vi "FlexRay_Analyze_signal_values.vi"(10 "TLibFLexRay":T2, 11 "DataBase_array":T1) -> (3 "data out":T3)   [LabVIEW 2014]
uses:
  Typedef/TDBProperties.ctl
  Typedef/TDBECUProperties.ctl
  Typedef/TDBFrameProperties.ctl
  Typedef/CAN/TCANSignal.ctl
  Typedef/LIN/TLINSignal.ctl
  Typedef/FlexRay/TFlexRaySignal.ctl
  Typedef/TDBSignalProperties.ctl
  FlexRay_Function/Typedef/TLibFLexRay.ctl
  Typedef/DataBase_array.ctl
  Typedef/DataBase_array_index.ctl
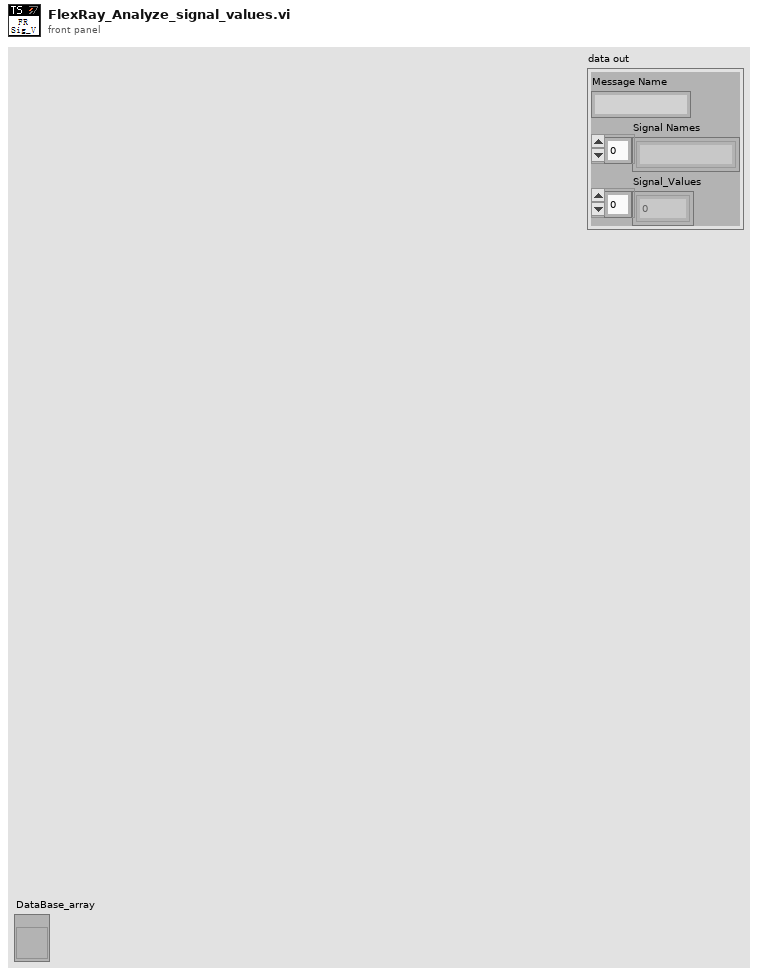
[diagram p1: front panel]
types:
  T1 = typedef "DataBase_array_index.ctl" = refnum<vi>
  T2 = typedef "TLibFLexRay.ctl" = cluster{"FIdxChn":u8, "FChannelMask":u8, "FDir":u8, "FPayloadLength":u8, "FActualPayloadLength":u8, "FCycleNumber":u8, "FCCType":u8, "FFrameType":u8, "FHeaderCRCA":u16, "FHeaderCRCB":u16, "FFrameStateInfo":u16, "FSlotId":u16, "FFrameFlags":u32, "FFrameCRC":u32, "FReserved1":u64, "FReserved2":u64, "FTimeUs":u64, "FData":cluster{"数值":u8, "数值 9":u8, "数值 17":u8, "数值 25":u8, "数值 33":u8, "数值 41":u8, "数值 49":u8, "数值 57":u8, "数值 65":u8, "数值 73":u8, "数值 81":u8, "数值 89":u8, "数值 97":u8, "数值 105":u8, "数值 98":u8, "数值 99":u8, "数值 2":u8, "数值 10":u8, "数值 18":u8, "数值 26":u8, "数值 34":u8, "数值 42":u8, "数值 50":u8, "数值 58":u8, "数值 66":u8, "数值 74":u8, "数值 82":u8, "数值 90":u8, "数值 100":u8, "数值 106":u8, "数值 101":u8, "数值 102":u8, "数值 3":u8, "数值 11":u8, "数值 19":u8, "数值 27":u8, "数值 35":u8, "数值 43":u8, "数值 51":u8, "数值 59":u8, "数值 67":u8, "数值 75":u8, "数值 83":u8, "数值 91":u8, "数值 103":u8, "数值 107":u8, "数值 104":u8, "数值 108":u8, "数值 4":u8, "数值 12":u8, "数值 20":u8, "数值 28":u8, "数值 36":u8, "数值 44":u8, "数值 52":u8, "数值 60":u8, "数值 68":u8, "数值 76":u8, "数值 84":u8, "数值 92":u8, "数值 109":u8, "数值 110":u8, "数值 111":u8, "数值 112":u8, "数值 5":u8, "数值 13":u8, "数值 21":u8, "数值 29":u8, "数值 37":u8, "数值 45":u8, "数值 53":u8, "数值 61":u8, "数值 69":u8, "数值 77":u8, "数值 85":u8, "数值 93":u8, "数值 113":u8, "数值 114":u8, "数值 115":u8, "数值 116":u8, "数值 6":u8, "数值 14":u8, "数值 22":u8, "数值 30":u8, "数值 38":u8, "数值 46":u8, "数值 54":u8, "数值 62":u8, "数值 70":u8, "数值 78":u8, "数值 86":u8, "数值 94":u8, "数值 117":u8, "数值 118":u8, "数值 119":u8, "数值 120":u8, "数值 7":u8, "数值 15":u8, "数值 23":u8, "数值 31":u8, "数值 39":u8, "数值 47":u8, "数值 55":u8, "数值 63":u8, "数值 71":u8, "数值 79":u8, "数值 87":u8, "数值 95":u8, "数值 121":u8, "数值 122":u8, "数值 123":u8, "数值 124":u8, "数值 8":u8, "数值 16":u8, "数值 24":u8, "数值 32":u8, "数值 40":u8, "数值 48":u8, "数值 56":u8, "数值 64":u8, "数值 72":u8, "数值 80":u8, "数值 88":u8, "数值 96":u8, "数值 125":u8, "数值 126":u8, "数值 127":u8, "数值 128":u8, "数值 129":u8, "数值 130":u8, "数值 131":u8, "数值 132":u8, "数值 133":u8, "数值 134":u8, "数值 135":u8, "数值 136":u8, "数值 137":u8, "数值 138":u8, "数值 139":u8, "数值 140":u8, "数值 141":u8, "数值 142":u8, "数值 143":u8, "数值 144":u8, "数值 145":u8, "数值 146":u8, "数值 147":u8, "数值 148":u8, "数值 149":u8, "数值 150":u8, "数值 151":u8, "数值 152":u8, "数值 153":u8, "数值 154":u8, "数值 155":u8, "数值 156":u8, "数值 157":u8, "数值 158":u8, "数值 159":u8, "数值 160":u8, "数值 161":u8, "数值 162":u8, "数值 163":u8, "数值 164":u8, "数值 165":u8, "数值 166":u8, "数值 167":u8, "数值 168":u8, "数值 169":u8, "数值 170":u8, "数值 171":u8, "数值 172":u8, "数值 173":u8, "数值 174":u8, "数值 175":u8, "数值 176":u8, "数值 177":u8, "数值 178":u8, "数值 179":u8, "数值 180":u8, "数值 181":u8, "数值 182":u8, "数值 183":u8, "数值 184":u8, "数值 185":u8, "数值 186":u8, "数值 187":u8, "数值 188":u8, "数值 189":u8, "数值 190":u8, "数值 191":u8, "数值 192":u8, "数值 193":u8, "数值 194":u8, "数值 195":u8, "数值 196":u8, "数值 197":u8, "数值 198":u8, "数值 199":u8, "数值 200":u8, "数值 201":u8, "数值 202":u8, "数值 203":u8, "数值 204":u8, "数值 205":u8, "数值 206":u8, "数值 207":u8, "数值 208":u8, "数值 209":u8, "数值 210":u8, "数值 211":u8, "数值 212":u8, "数值 213":u8, "数值 214":u8, "数值 215":u8, "数值 216":u8, "数值 217":u8, "数值 218":u8, "数值 219":u8, "数值 220":u8, "数值 221":u8, "数值 222":u8, "数值 223":u8, "数值 224":u8, "数值 225":u8, "数值 226":u8, "数值 227":u8, "数值 228":u8, "数值 229":u8, "数值 230":u8, "数值 231":u8, "数值 232":u8, "数值 233":u8, "数值 234":u8, "数值 235":u8, "数值 236":u8, "数值 237":u8, "数值 238":u8, "数值 239":u8, "数值 241":u8, "数值 242":u8, "数值 243":u8, "数值 244":u8, "数值 245":u8, "数值 246":u8, "数值 247":u8, "数值 248":u8, "数值 249":u8, "数值 250":u8, "数值 251":u8, "数值 252":u8, "数值 253":u8, "数值 254":u8, "数值 255":u8}}
  T3 = cluster{"Message Name":string, "Signal Names":string[], "Signal_Values":dbl[]}
  T4 = typedef "DataBase_array.ctl" = cluster{"db_properties":T5, "ECU_array":cluster{"TDBECUProperties":T6, "TX_Frame_array":cluster{"Frame_Properties":T7, "signal_array":T8[]}[], "RX_Frame_array":cluster{"Frame_Properties":T7, "signal_array":T8[]}[]}[]}[]
  T5 = typedef "TDBProperties.ctl" = cluster{"FDBIndex":i32, "FSignalCount":i32, "FFrameCount":i32, "FECUCount":i32, "FSupportedChannelMask":u64, "FName":cluster{"数值":u64, "数值 2":u64, "数值 3":u64, "数值 4":u64, "数值 5":u64, "数值 6":u64, "数值 7":u64, "数值 8":u64, "数值 9":u64, "数值 10":u64, "数值 11":u64, "数值 12":u64, "数值 13":u64, "数值 14":u64, "数值 15":u64, "数值 16":u64, "数值 17":u64, "数值 18":u64, "数值 19":u64, "数值 20":u64, "数值 21":u64, "数值 22":u64, "数值 23":u64, "数值 24":u64, "数值 25":u64, "数值 26":u64, "数值 27":u64, "数值 28":u64, "数值 29":u64, "数值 30":u64, "数值 31":u64, "数值 32":u64, "数值 33":u64, "数值 34":u64, "数值 35":u64, "数值 36":u64, "数值 37":u64, "数值 38":u64, "数值 39":u64, "数值 40":u64, "数值 41":u64, "数值 42":u64, "数值 43":u64, "数值 44":u64, "数值 45":u64, "数值 46":u64, "数值 47":u64, "数值 48":u64, "数值 49":u64, "数值 50":u64, "数值 51":u64, "数值 52":u64, "数值 53":u64, "数值 54":u64, "数值 55":u64, "数值 56":u64, "数值 57":u64, "数值 58":u64, "数值 59":u64, "数值 60":u64, "数值 61":u64, "数值 62":u64, "数值 63":u64, "数值 64":u64}, "FComment":cluster{"数值":u64, "数值 2":u64, "数值 3":u64, "数值 4":u64, "数值 5":u64, "数值 6":u64, "数值 7":u64, "数值 8":u64, "数值 9":u64, "数值 10":u64, "数值 11":u64, "数值 12":u64, "数值 13":u64, "数值 14":u64, "数值 15":u64, "数值 16":u64, "数值 17":u64, "数值 18":u64, "数值 19":u64, "数值 20":u64, "数值 21":u64, "数值 22":u64, "数值 23":u64, "数值 24":u64, "数值 25":u64, "数值 26":u64, "数值 27":u64, "数值 28":u64, "数值 29":u64, "数值 30":u64, "数值 31":u64, "数值 32":u64, "数值 33":u64, "数值 34":u64, "数值 35":u64, "数值 36":u64, "数值 37":u64, "数值 38":u64, "数值 39":u64, "数值 40":u64, "数值 41":u64, "数值 42":u64, "数值 43":u64, "数值 44":u64, "数值 45":u64, "数值 46":u64, "数值 47":u64, "数值 48":u64, "数值 49":u64, "数值 50":u64, "数值 51":u64, "数值 52":u64, "数值 53":u64, "数值 54":u64, "数值 55":u64, "数值 56":u64, "数值 57":u64, "数值 58":u64, "数值 59":u64, "数值 60":u64, "数值 61":u64, "数值 62":u64, "数值 63":u64, "数值 64":u64}, "FFlags":u32, "FDBId":u32}
  T6 = typedef "TDBECUProperties.ctl" = cluster{"FDBIndex":i32, "FECUIndex":i32, "FTxFrameCount":i32, "FRxFrameCount":i32, "FName":cluster{"数值":u64, "数值 2":u64, "数值 3":u64, "数值 4":u64, "数值 5":u64, "数值 6":u64, "数值 7":u64, "数值 8":u64, "数值 9":u64, "数值 10":u64, "数值 11":u64, "数值 12":u64, "数值 13":u64, "数值 14":u64, "数值 15":u64, "数值 16":u64, "数值 17":u64, "数值 18":u64, "数值 19":u64, "数值 20":u64, "数值 21":u64, "数值 22":u64, "数值 23":u64, "数值 24":u64, "数值 25":u64, "数值 26":u64, "数值 27":u64, "数值 28":u64, "数值 29":u64, "数值 30":u64, "数值 31":u64, "数值 32":u64, "数值 33":u64, "数值 34":u64, "数值 35":u64, "数值 36":u64, "数值 37":u64, "数值 38":u64, "数值 39":u64, "数值 40":u64, "数值 41":u64, "数值 42":u64, "数值 43":u64, "数值 44":u64, "数值 45":u64, "数值 46":u64, "数值 47":u64, "数值 48":u64, "数值 49":u64, "数值 50":u64, "数值 51":u64, "数值 52":u64, "数值 53":u64, "数值 54":u64, "数值 55":u64, "数值 56":u64, "数值 57":u64, "数值 58":u64, "数值 59":u64, "数值 60":u64, "数值 61":u64, "数值 62":u64, "数值 63":u64, "数值 64":u64}, "FComment":cluster{"数值":u64, "数值 2":u64, "数值 3":u64, "数值 4":u64, "数值 5":u64, "数值 6":u64, "数值 7":u64, "数值 8":u64, "数值 9":u64, "数值 10":u64, "数值 11":u64, "数值 12":u64, "数值 13":u64, "数值 14":u64, "数值 15":u64, "数值 16":u64, "数值 17":u64, "数值 18":u64, "数值 19":u64, "数值 20":u64, "数值 21":u64, "数值 22":u64, "数值 23":u64, "数值 24":u64, "数值 25":u64, "数值 26":u64, "数值 27":u64, "数值 28":u64, "数值 29":u64, "数值 30":u64, "数值 31":u64, "数值 32":u64, "数值 33":u64, "数值 34":u64, "数值 35":u64, "数值 36":u64, "数值 37":u64, "数值 38":u64, "数值 39":u64, "数值 40":u64, "数值 41":u64, "数值 42":u64, "数值 43":u64, "数值 44":u64, "数值 45":u64, "数值 46":u64, "数值 47":u64, "数值 48":u64, "数值 49":u64, "数值 50":u64, "数值 51":u64, "数值 52":u64, "数值 53":u64, "数值 54":u64, "数值 55":u64, "数值 56":u64, "数值 57":u64, "数值 58":u64, "数值 59":u64, "数值 60":u64, "数值 61":u64, "数值 62":u64, "数值 63":u64, "数值 64":u64}}
  T7 = typedef "TDBFrameProperties.ctl" = cluster{"FDBIndex":i32, "FECUIndex":i32, "FFrameIndex":i32, "FIsTx":u8, "FReserved1":u8, "FCycleTimeMs":u16, "TSignalType":i32, "FCANIsDataFrame":u8, "FCANIsStdFrame":u8, "FCANIsEdl":u8, "FCANIsBrs":u8, "FCANIdentifier":i32, "FCANDLC":i32, "FCANDataBytes":i32, "FLINIdentifier":i32, "FLINDLC":i32, "FFRChannelMask":u8, "FFRBaseCycle":u8, "FFRCycleRepetition":u8, "FFRIsStartupFrame":u8, "FFRSlotId":u16, "FFRDLC":u16, "FFRCycleMask":u64, "FSignalCount":i32, "FName":cluster{"数值":u64, "数值 2":u64, "数值 3":u64, "数值 4":u64, "数值 5":u64, "数值 6":u64, "数值 7":u64, "数值 8":u64, "数值 9":u64, "数值 10":u64, "数值 11":u64, "数值 12":u64, "数值 13":u64, "数值 14":u64, "数值 15":u64, "数值 16":u64, "数值 17":u64, "数值 18":u64, "数值 19":u64, "数值 20":u64, "数值 21":u64, "数值 22":u64, "数值 23":u64, "数值 24":u64, "数值 25":u64, "数值 26":u64, "数值 27":u64, "数值 28":u64, "数值 29":u64, "数值 30":u64, "数值 31":u64, "数值 32":u64, "数值 33":u64, "数值 34":u64, "数值 35":u64, "数值 36":u64, "数值 37":u64, "数值 38":u64, "数值 39":u64, "数值 40":u64, "数值 41":u64, "数值 42":u64, "数值 43":u64, "数值 44":u64, "数值 45":u64, "数值 46":u64, "数值 47":u64, "数值 48":u64, "数值 49":u64, "数值 50":u64, "数值 51":u64, "数值 52":u64, "数值 53":u64, "数值 54":u64, "数值 55":u64, "数值 56":u64, "数值 57":u64, "数值 58":u64, "数值 59":u64, "数值 60":u64, "数值 61":u64, "数值 62":u64, "数值 63":u64, "数值 64":u64}, "FComment":cluster{"数值":u64, "数值 2":u64, "数值 3":u64, "数值 4":u64, "数值 5":u64, "数值 6":u64, "数值 7":u64, "数值 8":u64, "数值 9":u64, "数值 10":u64, "数值 11":u64, "数值 12":u64, "数值 13":u64, "数值 14":u64, "数值 15":u64, "数值 16":u64, "数值 17":u64, "数值 18":u64, "数值 19":u64, "数值 20":u64, "数值 21":u64, "数值 22":u64, "数值 23":u64, "数值 24":u64, "数值 25":u64, "数值 26":u64, "数值 27":u64, "数值 28":u64, "数值 29":u64, "数值 30":u64, "数值 31":u64, "数值 32":u64, "数值 33":u64, "数值 34":u64, "数值 35":u64, "数值 36":u64, "数值 37":u64, "数值 38":u64, "数值 39":u64, "数值 40":u64, "数值 41":u64, "数值 42":u64, "数值 43":u64, "数值 44":u64, "数值 45":u64, "数值 46":u64, "数值 47":u64, "数值 48":u64, "数值 49":u64, "数值 50":u64, "数值 51":u64, "数值 52":u64, "数值 53":u64, "数值 54":u64, "数值 55":u64, "数值 56":u64, "数值 57":u64, "数值 58":u64, "数值 59":u64, "数值 60":u64, "数值 61":u64, "数值 62":u64, "数值 63":u64, "数值 64":u64}}
  T8 = typedef "TDBSignalProperties.ctl" = cluster{"FDBIndex":i32, "FECUIndex":i32, "FFrameIndex":i32, "FSignalIndex":i32, "FIsTx":u8, "FReserved1":u8, "FReserved2":u8, "FReserved3":u8, "TSignalType":i32, "TCANSignal":T9, "TLINSignal":T10, "TFlexRaySignal":T11, "FParentFrameId":i32, "FInitValue":dbl, "FName":cluster{"数值":u64, "数值 2":u64, "数值 3":u64, "数值 4":u64, "数值 5":u64, "数值 6":u64, "数值 7":u64, "数值 8":u64, "数值 9":u64, "数值 10":u64, "数值 11":u64, "数值 12":u64, "数值 13":u64, "数值 14":u64, "数值 15":u64, "数值 16":u64, "数值 17":u64, "数值 18":u64, "数值 19":u64, "数值 20":u64, "数值 21":u64, "数值 22":u64, "数值 23":u64, "数值 24":u64, "数值 25":u64, "数值 26":u64, "数值 27":u64, "数值 28":u64, "数值 29":u64, "数值 30":u64, "数值 31":u64, "数值 32":u64, "数值 33":u64, "数值 34":u64, "数值 35":u64, "数值 36":u64, "数值 37":u64, "数值 38":u64, "数值 39":u64, "数值 40":u64, "数值 41":u64, "数值 42":u64, "数值 43":u64, "数值 44":u64, "数值 45":u64, "数值 46":u64, "数值 47":u64, "数值 48":u64, "数值 49":u64, "数值 50":u64, "数值 51":u64, "数值 52":u64, "数值 53":u64, "数值 54":u64, "数值 55":u64, "数值 56":u64, "数值 57":u64, "数值 58":u64, "数值 59":u64, "数值 60":u64, "数值 61":u64, "数值 62":u64, "数值 63":u64, "数值 64":u64}, "FComment":cluster{"数值":u64, "数值 2":u64, "数值 3":u64, "数值 4":u64, "数值 5":u64, "数值 6":u64, "数值 7":u64, "数值 8":u64, "数值 9":u64, "数值 10":u64, "数值 11":u64, "数值 12":u64, "数值 13":u64, "数值 14":u64, "数值 15":u64, "数值 16":u64, "数值 17":u64, "数值 18":u64, "数值 19":u64, "数值 20":u64, "数值 21":u64, "数值 22":u64, "数值 23":u64, "数值 24":u64, "数值 25":u64, "数值 26":u64, "数值 27":u64, "数值 28":u64, "数值 29":u64, "数值 30":u64, "数值 31":u64, "数值 32":u64, "数值 33":u64, "数值 34":u64, "数值 35":u64, "数值 36":u64, "数值 37":u64, "数值 38":u64, "数值 39":u64, "数值 40":u64, "数值 41":u64, "数值 42":u64, "数值 43":u64, "数值 44":u64, "数值 45":u64, "数值 46":u64, "数值 47":u64, "数值 48":u64, "数值 49":u64, "数值 50":u64, "数值 51":u64, "数值 52":u64, "数值 53":u64, "数值 54":u64, "数值 55":u64, "数值 56":u64, "数值 57":u64, "数值 58":u64, "数值 59":u64, "数值 60":u64, "数值 61":u64, "数值 62":u64, "数值 63":u64, "数值 64":u64}}
  T9 = typedef "TCANSignal.ctl" = cluster{"FCANSgnType":u8, "FIsIntel":u8, "FStartBit":i32, "FLength":i32, "FFactor":dbl, "FOffset":dbl}
  T10 = typedef "TLINSignal.ctl" = cluster{"FLINSgnType":u8, "FIsIntel":u8, "FStartBit":i32, "FLength":i32, "FFactor":dbl, "FOffset":dbl}
  T11 = typedef "TFlexRaySignal.ctl" = cluster{"FFRSgnType":u8, "FCompuMethod":u8, "FReserved":u8, "FIsIntel":u8, "FStartBit":i32, "FUpdateBit":i32, "FLength":i32, "FFactor":dbl, "FOffset":dbl, "FActualStartBit":i32, "FActualUpdateBit":i32}
  T12 = cluster{"TDBECUProperties":T6, "TX_Frame_array":cluster{"Frame_Properties":T7, "signal_array":T8[]}[], "RX_Frame_array":cluster{"Frame_Properties":T7, "signal_array":T8[]}[]}[]
  T13 = cluster{"Frame_Properties":T7, "signal_array":T8[]}[]
  T14 = cluster{"数值":u8, "数值 9":u8, "数值 17":u8, "数值 25":u8, "数值 33":u8, "数值 41":u8, "数值 49":u8, "数值 57":u8, "数值 65":u8, "数值 73":u8, "数值 81":u8, "数值 89":u8, "数值 97":u8, "数值 105":u8, "数值 98":u8, "数值 99":u8, "数值 2":u8, "数值 10":u8, "数值 18":u8, "数值 26":u8, "数值 34":u8, "数值 42":u8, "数值 50":u8, "数值 58":u8, "数值 66":u8, "数值 74":u8, "数值 82":u8, "数值 90":u8, "数值 100":u8, "数值 106":u8, "数值 101":u8, "数值 102":u8, "数值 3":u8, "数值 11":u8, "数值 19":u8, "数值 27":u8, "数值 35":u8, "数值 43":u8, "数值 51":u8, "数值 59":u8, "数值 67":u8, "数值 75":u8, "数值 83":u8, "数值 91":u8, "数值 103":u8, "数值 107":u8, "数值 104":u8, "数值 108":u8, "数值 4":u8, "数值 12":u8, "数值 20":u8, "数值 28":u8, "数值 36":u8, "数值 44":u8, "数值 52":u8, "数值 60":u8, "数值 68":u8, "数值 76":u8, "数值 84":u8, "数值 92":u8, "数值 109":u8, "数值 110":u8, "数值 111":u8, "数值 112":u8, "数值 5":u8, "数值 13":u8, "数值 21":u8, "数值 29":u8, "数值 37":u8, "数值 45":u8, "数值 53":u8, "数值 61":u8, "数值 69":u8, "数值 77":u8, "数值 85":u8, "数值 93":u8, "数值 113":u8, "数值 114":u8, "数值 115":u8, "数值 116":u8, "数值 6":u8, "数值 14":u8, "数值 22":u8, "数值 30":u8, "数值 38":u8, "数值 46":u8, "数值 54":u8, "数值 62":u8, "数值 70":u8, "数值 78":u8, "数值 86":u8, "数值 94":u8, "数值 117":u8, "数值 118":u8, "数值 119":u8, "数值 120":u8, "数值 7":u8, "数值 15":u8, "数值 23":u8, "数值 31":u8, "数值 39":u8, "数值 47":u8, "数值 55":u8, "数值 63":u8, "数值 71":u8, "数值 79":u8, "数值 87":u8, "数值 95":u8, "数值 121":u8, "数值 122":u8, "数值 123":u8, "数值 124":u8, "数值 8":u8, "数值 16":u8, "数值 24":u8, "数值 32":u8, "数值 40":u8, "数值 48":u8, "数值 56":u8, "数值 64":u8, "数值 72":u8, "数值 80":u8, "数值 88":u8, "数值 96":u8, "数值 125":u8, "数值 126":u8, "数值 127":u8, "数值 128":u8, "数值 129":u8, "数值 130":u8, "数值 131":u8, "数值 132":u8, "数值 133":u8, "数值 134":u8, "数值 135":u8, "数值 136":u8, "数值 137":u8, "数值 138":u8, "数值 139":u8, "数值 140":u8, "数值 141":u8, "数值 142":u8, "数值 143":u8, "数值 144":u8, "数值 145":u8, "数值 146":u8, "数值 147":u8, "数值 148":u8, "数值 149":u8, "数值 150":u8, "数值 151":u8, "数值 152":u8, "数值 153":u8, "数值 154":u8, "数值 155":u8, "数值 156":u8, "数值 157":u8, "数值 158":u8, "数值 159":u8, "数值 160":u8, "数值 161":u8, "数值 162":u8, "数值 163":u8, "数值 164":u8, "数值 165":u8, "数值 166":u8, "数值 167":u8, "数值 168":u8, "数值 169":u8, "数值 170":u8, "数值 171":u8, "数值 172":u8, "数值 173":u8, "数值 174":u8, "数值 175":u8, "数值 176":u8, "数值 177":u8, "数值 178":u8, "数值 179":u8, "数值 180":u8, "数值 181":u8, "数值 182":u8, "数值 183":u8, "数值 184":u8, "数值 185":u8, "数值 186":u8, "数值 187":u8, "数值 188":u8, "数值 189":u8, "数值 190":u8, "数值 191":u8, "数值 192":u8, "数值 193":u8, "数值 194":u8, "数值 195":u8, "数值 196":u8, "数值 197":u8, "数值 198":u8, "数值 199":u8, "数值 200":u8, "数值 201":u8, "数值 202":u8, "数值 203":u8, "数值 204":u8, "数值 205":u8, "数值 206":u8, "数值 207":u8, "数值 208":u8, "数值 209":u8, "数值 210":u8, "数值 211":u8, "数值 212":u8, "数值 213":u8, "数值 214":u8, "数值 215":u8, "数值 216":u8, "数值 217":u8, "数值 218":u8, "数值 219":u8, "数值 220":u8, "数值 221":u8, "数值 222":u8, "数值 223":u8, "数值 224":u8, "数值 225":u8, "数值 226":u8, "数值 227":u8, "数值 228":u8, "数值 229":u8, "数值 230":u8, "数值 231":u8, "数值 232":u8, "数值 233":u8, "数值 234":u8, "数值 235":u8, "数值 236":u8, "数值 237":u8, "数值 238":u8, "数值 239":u8, "数值 241":u8, "数值 242":u8, "数值 243":u8, "数值 244":u8, "数值 245":u8, "数值 246":u8, "数值 247":u8, "数值 248":u8, "数值 249":u8, "数值 250":u8, "数值 251":u8, "数值 252":u8, "数值 253":u8, "数值 254":u8, "数值 255":u8}
  T15 = cluster{"数值":u64, "数值 2":u64, "数值 3":u64, "数值 4":u64, "数值 5":u64, "数值 6":u64, "数值 7":u64, "数值 8":u64, "数值 9":u64, "数值 10":u64, "数值 11":u64, "数值 12":u64, "数值 13":u64, "数值 14":u64, "数值 15":u64, "数值 16":u64, "数值 17":u64, "数值 18":u64, "数值 19":u64, "数值 20":u64, "数值 21":u64, "数值 22":u64, "数值 23":u64, "数值 24":u64, "数值 25":u64, "数值 26":u64, "数值 27":u64, "数值 28":u64, "数值 29":u64, "数值 30":u64, "数值 31":u64, "数值 32":u64, "数值 33":u64, "数值 34":u64, "数值 35":u64, "数值 36":u64, "数值 37":u64, "数值 38":u64, "数值 39":u64, "数值 40":u64, "数值 41":u64, "数值 42":u64, "数值 43":u64, "数值 44":u64, "数值 45":u64, "数值 46":u64, "数值 47":u64, "数值 48":u64, "数值 49":u64, "数值 50":u64, "数值 51":u64, "数值 52":u64, "数值 53":u64, "数值 54":u64, "数值 55":u64, "数值 56":u64, "数值 57":u64, "数值 58":u64, "数值 59":u64, "数值 60":u64, "数值 61":u64, "数值 62":u64, "数值 63":u64, "数值 64":u64}
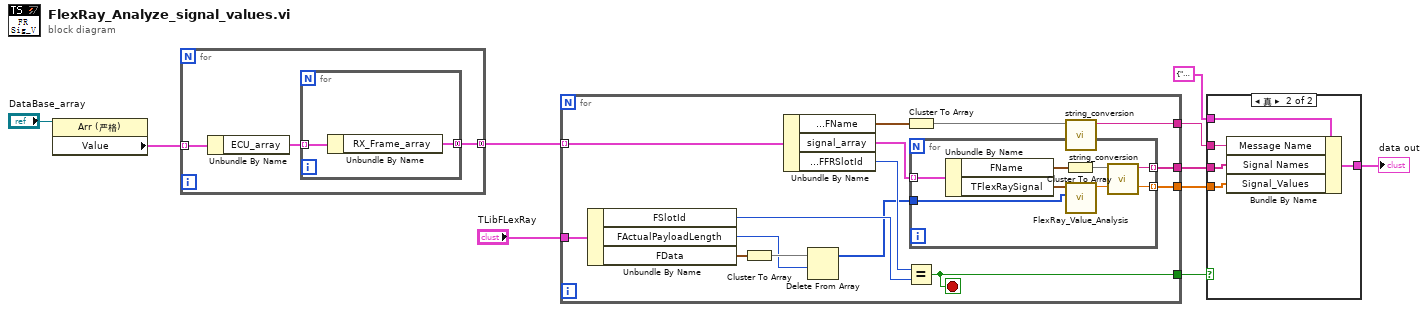
[diagram p0: block diagram]
diagram:
  n1 = property class="Arr (严格)"(reference="DataBase_array") -> ("Value"=w1:T4)  [unwired: 1 in, 2 out]
  n2 = for {
    tunnel: w1 -> [w13] mode=indexing
    tunnel: [w11] -> w10 mode=concatenating
    n3 = Unbundle By Name(w13) -> ("ECU_array"=w12:T12)
    n4 = for {
      tunnel: w12 -> [w15] mode=indexing
      tunnel: [w14] -> w11 mode=concatenating
      n5 = Unbundle By Name(w15) -> ("RX_Frame_array"=w14:T13)
    }
  }
  n6 = for {
    tunnel: w10 -> [w30] mode=indexing
    tunnel: "TLibFLexRay" -> [w26]
    tunnel: [w23] -> w9
    tunnel: [w22] -> w8
    tunnel: [w17] -> w4
    tunnel: [w16] -> w3
    stop <- w16 stop-if-true
    n7 = Unbundle By Name(w26) -> ("FSlotId"=w25:u16, "FActualPayloadLength"=w19:u8, "FData"=w21:T14)
    n8 = Cluster To Array(cluster=w21) -> (array=w20:u8[])
    n9 = Unbundle By Name(w30) -> ("Frame_Properties.FName"=w28:T15, "signal_array"=w27:T8[], "Frame_Properties.FFRSlotId"=w24:u16)
    n10 = Delete From Array(array=w20, length=w19) -> (array with subset deleted=w18:u8[])  [unwired: 1 in, 1 out]
    n11 = Cluster To Array(cluster=w28) -> (array=w29:u64[])
    n12 = Equal?(x=w24, y=w25) -> (x = y?=w16:bool)
    n13 = for {
      tunnel: w27 -> [w37] mode=indexing
      tunnel: [w34] -> w22 mode=indexing
      tunnel: w18 -> [w32]
      tunnel: [w31] -> w17 mode=indexing
      n14 = Unbundle By Name(w37) -> ("FName"=w36:T15, "TFlexRaySignal"=w33:T11)
      n15 = Cluster To Array(cluster=w36) -> (array=w35:u64[])
      n16 = call "FlexRay_Value_Analysis.vi"("FDatas"=w32, "TFlexRaySignal"=w33) -> ("Signal Value"=w31:dbl)  [unwired: 9 in]
      n17 = call "string_conversion.vi"("FName"=w35) -> ("string"=w34:string)  [unwired: 10 in]
    }
    n18 = call "string_conversion.vi"("FName"=w29) -> ("string"=w23:string)  [unwired: 10 in]
  }
  n19 = case shown="真" w3 {
    tunnel: w9 -> [_ w43]
    tunnel: w8 -> [_ w42]
    tunnel: [w38 w41] -> w7
    tunnel: T3 {"Message Name"="", "Signal Names"=[], "Signal_Values"=[]} ("data out") -> [w38 w40]
    tunnel: w4 -> [_ w39]
    frame False {
    }
    frame True {
      n20 = Bundle By Name(cluster=w40, "Message Name"=w43, "Signal Names"=w42, "Signal_Values"=w39) -> (w41:T3)
    }
  }
  "data out" <- w7
